vi "Vol-Get master frames number.vi"(7 "Source number of frames":T1(ring), 8 "error in (no error)":errorcluster) -> (0 "error out":errorcluster, 1 "Number of Frames":u32, 2 "Cancelled due to the selected \nAVI file being located within an\n\"Exported 8-bit videos\" directory!":bool, 5 "Reinitialising in AVI1 mode":bool)   [LabVIEW 2017]
uses:
  Functional Imaging Viewer/SubVIs/Experiment header interface/Typedefs/Header file interface module functions enum.ctl
  Functional Imaging Viewer/Typedefs/Get-Set-Clear Control.ctl
  Timelapse Viewer/Globals/gl_Time series viewer globals.vi
  Functional Imaging Viewer/SubVIs/Experiment header interface/Typedefs/Header file type enum.ctl
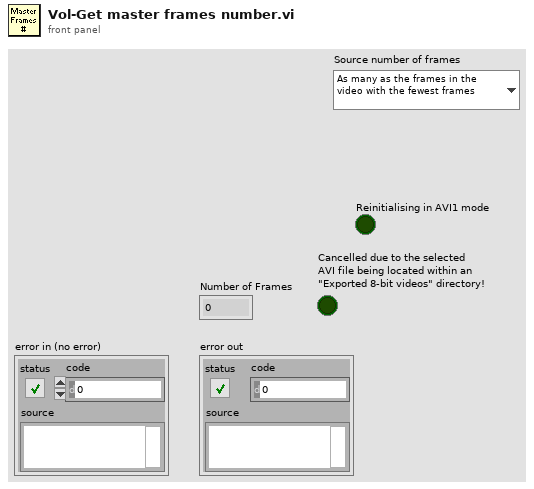
[diagram p1: front panel]
types:
  T1 = enum16{"As many as the frames in the video with the fewest frames", "As many as the number of cycles"}
  T2 = typedef "Header file interface module functions enum.ctl" = enum16{"Load experiment header file", "Save experiment header file", "Clear stored values", "Read stored values", "Update specific value in memory", "Update values in memory"}
  T3 = typedef "Get-Set-Clear Control.ctl" = enum16{"Get", "Set", "Clear"}
  T4 = typedef "Time series viewer refs.ctl" = cluster{"This VI":refnum<vi>, "Image control":refnum<vi>, "AVI Mode ind":refnum<vi>, "Play":refnum<vi>, "Stop":refnum<vi>, "Back":refnum<vi>, "Scrollbar":refnum<vi>, "Video length info":refnum<vi>, "Expected speed values":refnum<vi>, "Intensity":refnum<vi>, "Path":refnum<vi>, "Selection sliders":refnum<vi>, "Speed Graph ref":refnum<vi>, "Frame rate set (fps)":refnum<vi>, "Channel to load":refnum<vi>, "Number of rows to generate":refnum<vi>, "Colour":refnum<vi>}
  T5 = typedef "Header parameters cluster-ALL.ctl" = cluster{"LOGIN":T6, "GLOBAL PARAMETERS":T7, "IMAGING MODES":T9, "TIME SERIES":T10, "MOTOR Z-STACK ":T13, "AOL Z-STACK":T14, "FUNCTIONAL IMAGING":T15, "MOVEMENT CORRECTION":T19, "CALIBRATION":T21, "STATISTICS":T22, "BIOLOGY INFORMATION":T23}
  T6 = typedef "Header params -Login.ctl" = cluster{"User":string, "Profile":string, "Software Version":string, "Experiment Date Time":timestamp}
  T7 = typedef "Header params-Global Parameters.ctl" = cluster{"MicroscopeID":string, "Microscope Type":string, "Objective":string, "Field of View (um)":dbl, "Fill time (us)":dbl, "Experiment Type":T8, "Stimuli Trigger":bool, "Speed Logging":bool}
  T8 = typedef "Experiment Type.ctl" = enum16{"In vivo", "In vitro", "Testing", "Calibration", "Other"}
  T9 = typedef "Header params-Imaging Modes.ctl" = cluster{"Time Series":bool, "Motor Zstack":bool, "AOL Zstack":bool, "Functional Imaging":bool}
  T10 = typedef "Header params-Time Series.ctl" = cluster{"Basic Image meta data":T11, "AOL z":dbl}
  T11 = typedef "Header params-Basic image meta data.ctl" = cluster{"Wavelength (nm)":dbl, "# averaged frames":dbl, "laser power (%)":dbl, "Pockels":dbl, "pixel dwell time (us)":dbl, "pmt 1":dbl, "pmt 2":dbl, "back apperture":dbl, "zoom":dbl, "field of view":dbl, "Frame Size":T12, "AOL x centre":dbl, "AOL y centre":dbl, "Stage x position":dbl, "Stage y position":dbl, "Stage z position":dbl}
  T12 = typedef "Frame Size.ctl" = u16
  T13 = typedef "Header params-Motor Z-stack.ctl" = cluster{"Hdr Basic Image meta data":T11, "Z Start":dbl, "Z Stop":dbl, "No of Planes":i32}
  T14 = typedef "Header params-AOL Z-stack.ctl" = cluster{"Hdr Basic Image meta data":T11, "Z Start":dbl, "Z Stop":dbl, "No of Planes":i32}
  T15 = typedef "Header params-Functional Imaging.ctl" = cluster{"Functional Mode":T16, "Pockels Modulation":bool, "Number of pois":dbl, "Number of miniscans":dbl, "Number of cycles":dbl, "Number of trials":dbl, "Miniscan dwell time per pixel (us)":dbl, "Number of pixels in miniscan":dbl, "poi dwell time":dbl, "Rectangle ROI length":dbl, "Rectangle ROI height":dbl, "AOL Mode":T17, "Plane Mode":T18, "video length (sec)":dbl, "Frame rate (fps)":dbl, "Stimuli Timing (usec)":dbl, "Acquisition Length":dbl, "Basic Image meta data":T11, "Z Start (um)":dbl, "Z Stop (um)":dbl}
  T16 = typedef "Functional Mode.ctl" = enum16{"Point", "Line", "Patch", "Plane", "Volume"}
  T17 = typedef "AOL modes.ctl" = enum16{"Raster", "Structural", "Pointing", "Mini Scan", "Alignment"}
  T18 = typedef "Plane Mode.ctl" = u16
  T19 = typedef "Header params-Movement correction.ctl" = cluster{"Movement Correction":bool, "Axial Reference":bool, "Reference X Pixels":dbl, "Reference Y Pixels":dbl, "Reference Source":T20, "Reference dwell time (us)":dbl, "Number of Z lines":dbl, "Size of Z pixels":dbl, "Axial Pixels":dbl, "Reference Zoom":dbl, "Reference Average":dbl, "Proportional Scale":dbl, "Integral Scale":dbl, "Proportional Scale Z":dbl, "Integral Scale Z":dbl, "Scan Interval":dbl, "Ref Plot Refresh Rate":dbl}
  T20 = typedef "Reference source.ctl" = enum16{"Green channel", "Red channel"}
  T21 = typedef "Header params-Calibration Setup.ctl" = cluster{"Pockels Calibration File":path, "Calibration_ini file":path, "Setup_ini file":path}
  T22 = typedef "Header params-statistics.ctl" = cluster{"Z-stack duration (sec)":dbl, "Number of acquired data-points":dbl, "Acquisition time (ms)":dbl, "Number of acquired frames":dbl}
  T23 = typedef "Biology Information.ctl" = cluster{"Animal Code or Name":string, "Animal DoB":string, "Animal Age":string, "Animal Sex":string, "Animal Weight":string, "Date of Injection":string, "Date of Implant":string, "Site of Injection":string, "Animal Ear Notch":string, "AAV constructs":string, "Genetic background":string, "Optical reporter":string, "Region of brain imaged":string, "Other \ncomments":string}
  T24 = typedef "Number of frames and locations cluster.ctl" = cluster{"Original number of frames":i32, "Number of valid frames":i32, "Frame number":i64[], "Frame location":i64[], "Frame rel.time":i64[]}
  T25 = typedef "Header file type enum.ctl" = enum16{"All parameters", "Params for funct acq w ROI or mscn", "Params for funct acq w rectangles", "Live imaging header parameters", "AOL Parameters"}
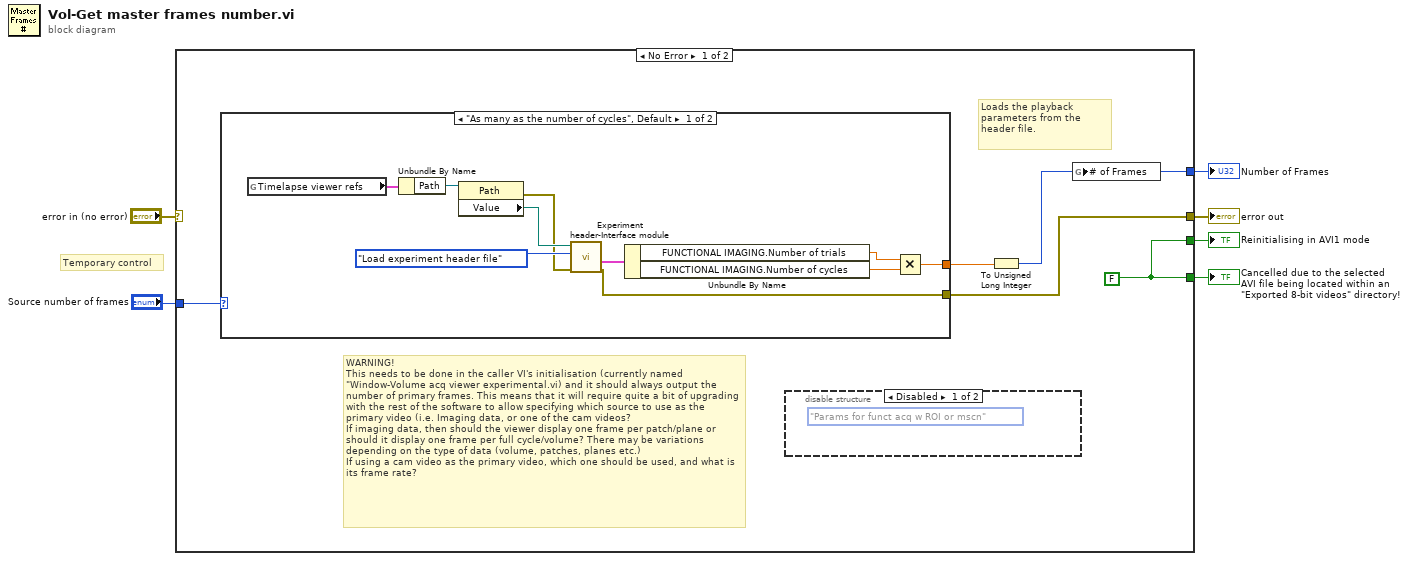
[diagram p0: block diagram]
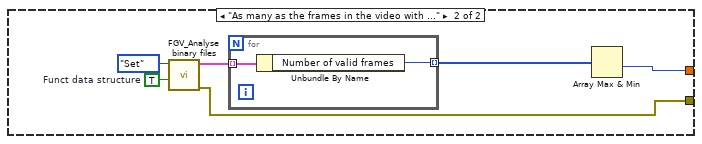
[diagram p3: hidden frame]
diagram:
  # "Temporary control"
  n1 = case shown="No Error" "error in (no error)" {
    selector: "error in (no error)" -> [_ w30]
    tunnel: [w9 w30] -> w6
    tunnel: [w7 _] -> w5
    tunnel: [w11 _] -> w3
    tunnel: [w11 _] -> w2
    tunnel: "Source number of frames" -> [w10 _]
    frame No Error {
      w11 = FALSE
      # "WARNING!\nThis needs to be done in the caller VI's initialisation (currently named \"Window-Volume acq viewer experimental.vi) and it should always output the number of primary frames. This means that it will require quite a bit of upgrading with the rest of the software to allow specifying which source to use as the primary video (i.e. Imaging data, or one of the cam videos? \nIf imaging data, then should the viewer display one frame per patch/plane or should it display one frame per full cycle/volume? There may be variations depending on the type of data (volume, patches, planes etc.) \nIf using a cam video as the primary video, which one should be used, and what is its frame rate?"
      # "Loads the playback parameters from the  header file."
      n2 = case shown="\"As many as the number of cycles\", Default" w10 {
        tunnel: [w12 w27] -> w8
        tunnel: [w15 w22] -> w9
        frame "As many as the number of cycles", Default {
          n3 = global read "gl_Time series viewer globals.vi" "Timelapse viewer refs"() -> (w19:T4)
          n4 = Unbundle By Name(w19) -> ("Path"=w18:refnum<vi>)
          n5 = property class="Path"(reference=w18) -> (error out=w16:errorcluster, "Value"=w17:path)  [unwired: 1 in, 1 out]
          n6 = call "Experiment header-Interface module.vi"("error in (no error)"=w16, "Function"=Header_file_interface_module_functions_enum."Load experiment header file", "Experiment data folder path"=w17) -> ("error out"=w15:errorcluster, "All header parameters out"=w21:T5)  [unwired: 7 in]
          n7 = Unbundle By Name(w21) -> ("FUNCTIONAL IMAGING.Number of trials"=w14:dbl, "FUNCTIONAL IMAGING.Number of cycles"=w13:dbl)
          n8 = Multiply(x=w14, y=w13) -> (x*y=w12:dbl)
        }
        frame "As many as the frames in the video with the fewest frames" {
          w23 = TRUE  # Funct data structure
          n9 = call "FGV_Analyse binary files.vi"("Funct data structure"=w23, "Get/Set info & refs"=Get-Set-Clear_Control."Set") -> ("Error out"=w22:errorcluster, "Frame numbers & locations in each video file"=w25:T24[])  [unwired: 6 in, 2 out]
          n10 = for {
            tunnel: w25 -> [w29] mode=indexing
            tunnel: [w28] -> w24 mode=indexing
            n11 = Unbundle By Name(w29) -> ("Number of valid frames"=w28:i32)
          }
          n12 = Array Max & Min(array=w24) -> (min value=w27:i32)  [unwired: 3 out]
        }
      }
      n13 = disable-structure shown="Disabled" {
        frame Disabled {
          (unwired) Header_file_type_enum."Params for funct acq w ROI or mscn" ("Header file type")
        }
        frame Enabled {
        }
      }
      n14 = To Unsigned Long Integer(number=w8) -> (unsigned 32bit integer=w7:u32)
      n15 = global write "gl_Time series viewer globals.vi" "# of Frames"(w7) -> ()
    }
    frame Error {
    }
  }
  "error out" <- w6
  "Number of Frames" <- w5
  "Reinitialising in AVI1 mode" <- w3
  "Cancelled due to the selected \nAVI file being located within an\n\"Exported 8-bit videos\" directory!" <- w2
